vi "CH1_write_byte_data_and_sign_into_mem_no_g_Rev01.vi"(0 "MB data":u8, 1 "UB data":u8, 3 "Address of the sign":string, 4 "USB Interface Name":refnum<visa-resource-name>="COM3", 5 "HB data":u8, 7 "LB data":u8, 8 "MB address":string, 9 "HB address":string, 11 "LB address":string, 12 "Sign Value":dbl, 13 "WRITE DATA":bool, 14 "Input buffer size":u32=16384, 16 "UB address":string, 17 "error in (no error)":errorcluster, 23 "Enable memory wright":bool) -> (18 "Reply 1":string, 19 "Reply 4":string, 20 "MB data string":string, 21 "UB data string":string, 22 "Reply 2":string, 24 "error out":errorcluster, 25 "HB data string":string, 26 "Reply 3":string, 27 "LB data string":string)   [LabVIEW 2012]
panel:
  out "T command Bytes sent 5":dbl
  out "T command Bytes sent 4":dbl
  out "T command Bytes sent 3":dbl
  out "T command Bytes sent 2":dbl
  out "T command Bytes sent":dbl
  out "First 'T' Number of bytes written":dbl
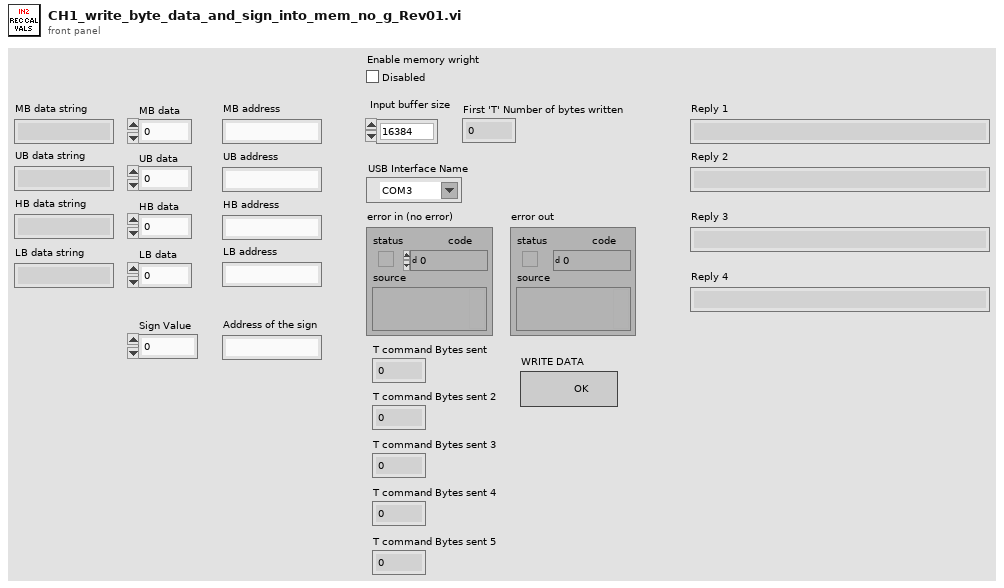
[diagram p1: front panel]
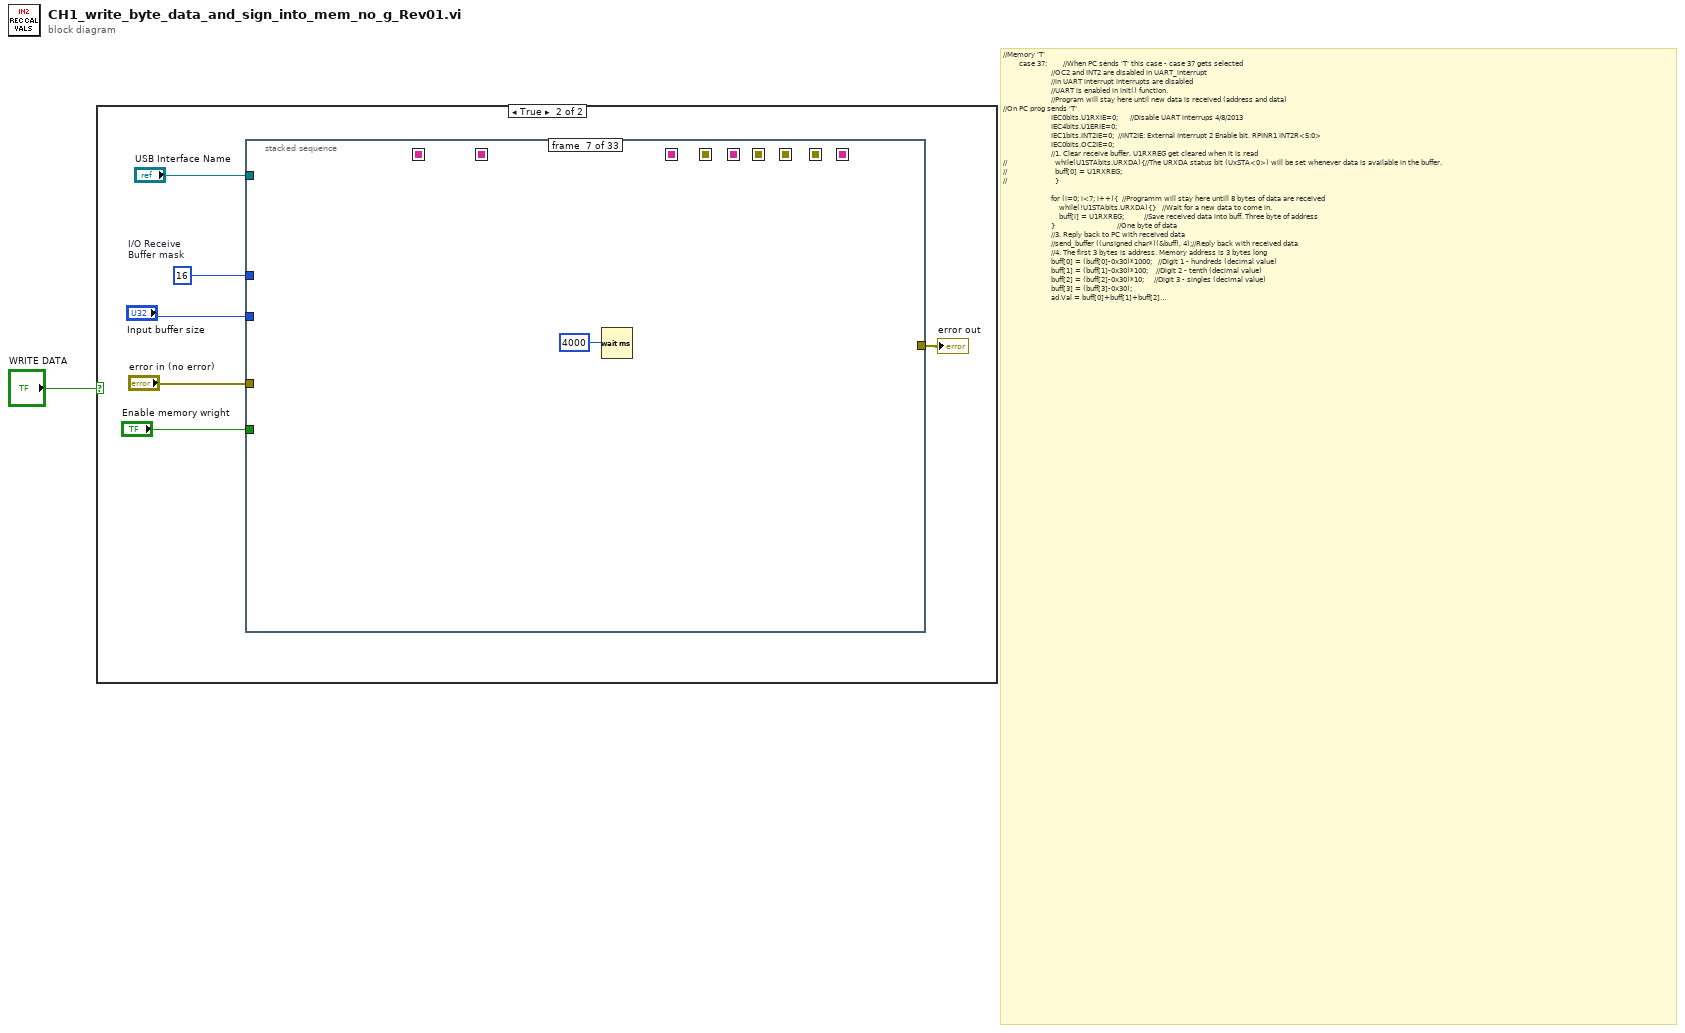
[diagram p0: block diagram]
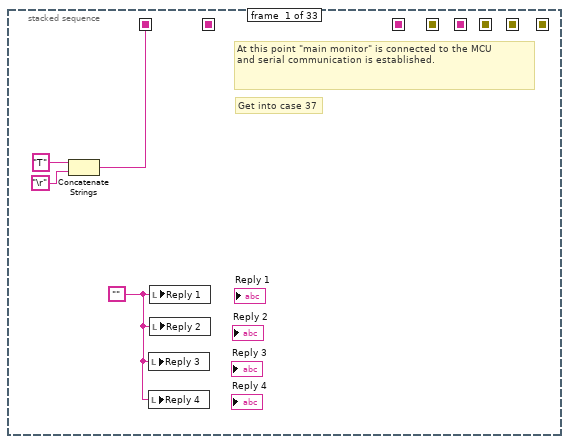
[diagram p3: hidden frame]
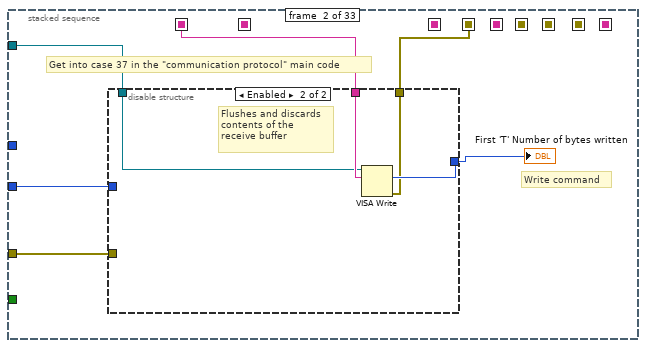
[diagram p4: hidden frame]
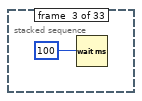
[diagram p6: hidden frame]
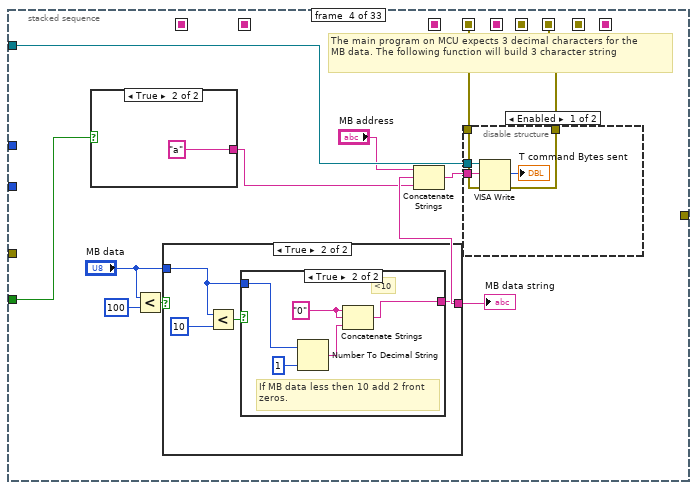
[diagram p7: hidden frame]
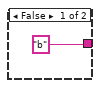
[diagram p8: hidden frame]
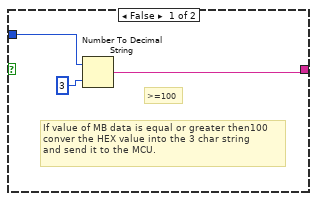
[diagram p9: hidden frame]
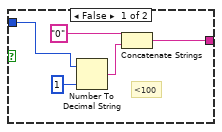
[diagram p10: hidden frame]
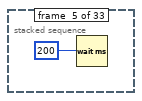
[diagram p12: hidden frame]
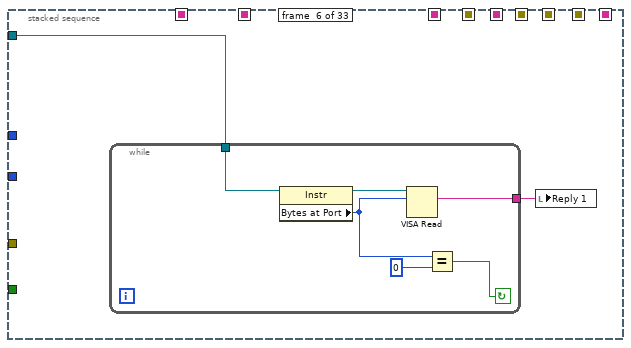
[diagram p13: hidden frame]
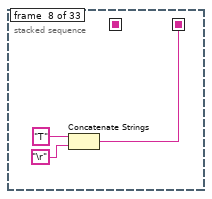
[diagram p14: hidden frame]
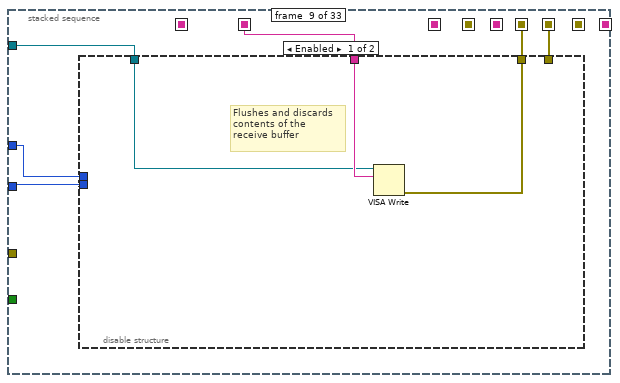
[diagram p15: hidden frame]
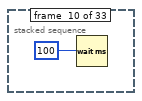
[diagram p17: hidden frame]
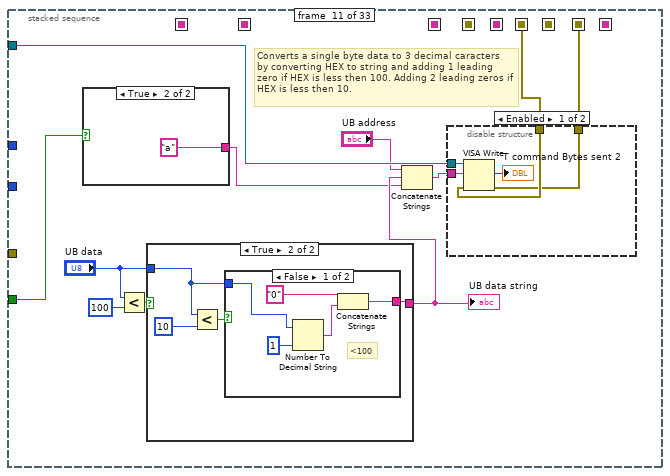
[diagram p18: hidden frame]
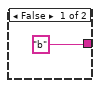
[diagram p19: hidden frame]
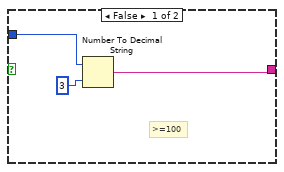
[diagram p20: hidden frame]
diagram:
  # "//Memory 'T'\n        case 37:        //When PC sends 'T' this case - case 37 gets selected\n                        //OC2 and INT2 are disabled in UART_interrupt\n                        //in UART interrupt interrupts are disabled\n                        //UART is enabled in init() function.\n                        //Program will stay here until new data is received (address and data)\n//On PC prog sends 'T'\n                        IEC0bits.U1RXIE=0;      //Disable UART interrups 4/8/2013\n                        IEC4bits.U1ERIE=0;\n                        IEC1bits.INT2IE=0;  //INT2IE: External Interrupt 2 Enable bit. RPINR1 INT2R<5:0>\n                        IEC0bits.OC2IE=0;\n                        //1. Clear receive buffer. U1RXREG get cleared when it is read\n//                        while(U1STAbits.URXDA){//The URXDA status bit (UxSTA<0>) will be set whenever data is available in the buffer.\n//                        buff[0] = U1RXREG;\n//                        }\n\n                        for (i=0; i<7; i++){  //Programm will stay here untill 8 bytes of data are received\n                            while(!U1STAbits.URXDA){}   //Wait for a new data to come in.\n                            buff[i] = U1RXREG;          //Save received data into buff. Three byte of address\n                        }                               //One byte of data\n                        //3. Reply back to PC with received data\n                        //send_buffer ((unsigned char*)(&buff), 4);//Reply back with received data\n                        //4. The first 3 bytes is address. Memory address is 3 bytes long\n                        buff[0] = (buff[0]-0x30)*1000;   //Digit 1 - hundreds (decimal value)\n                        buff[1] = (buff[1]-0x30)*100;    //Digit 2 - tenth (decimal value)\n                        buff[2] = (buff[2]-0x30)*10;     //Digit 3 - singles (decimal value)\n                        buff[3] = (buff[3]-0x30);\n                        ad.Val = buff[0]+buff[1]+buff[2]+buff[3];\n//                        send_char((char) ad.byte.MB);\n//                        send_char((char) ad.byte.UB);\n//                        send_char((char) ad.byte.HB);\n//                        send_char((char) ad.byte.LB); \n                        //5. The last 3 bytes are data\n                        buff[4] = buff[4]-0x30;//Load data. Byte number 4 is the data byte\n                        buff[5] = buff[5]-0x30;\n                        buff[6] = buff[6]-0x30;\n                        data = buff[4]*100+buff[5]*10+buff[6]; //Decimal value of 3 char digits\n                        //send_buffer ((unsigned char*)(&ad), 3);//Send back the received address\n                        //Erase byte by writing FFH into the address\n                        DF_WriteProtectDisable();   //Enable write to memory\n                        DF_IsBusy();                //Wait until the operation is done\n                        DF_WriteByte(ad.Val, data); //Write data into ad\n                        DF_IsBusy();\n                        DF_WriteDisable();          //Disable write\n                        DF_IsBusy();                        \n                        data=DF_ReadByte(ad.Val);     //4/22/13 return BYTE data\n//                       send_char((char) data);              //Read the memory location and reply with previously sent data\n//                        //Memory address for sign\n//                        buff[7] = (buff[7]-0x30)*1000;   //Digit 1 - hundreds (decimal value)\n//                        buff[8] = (buff[8]-0x30)*100;    //Digit 2 - tenth (decimal value)\n//                        buff[9] = (buff[9]-0x30)*10;     //Digit 3 - singles (decimal value)\n//                        buff[10] = (buff[10]-0x30);\n//                        ad.Val = buff[7]+buff[8]+buff[9]+buff[10];\n//                        //sign\n//                        sgn = buff[11];//<12\n                        \n                        selection = 1;\n                        rx_function=0; //4/11/13\n                        IEC0bits.U1RXIE=1;      //Reinable UART interrups\n                        IEC4bits.U1ERIE=1;                        \n                        IEC1bits.INT2IE=1;  //INT2IE: External Interrupt 2 Enable bit. RPINR1 INT2R<5:0>\n                        IEC0bits.OC2IE=1;\n                        \n\n            break;"
  n1 = case shown="True" "WRITE DATA" {
    frame False {
    }
    frame True {
      w5 = u16 16  # I/O Receive Buffer mask
      n2 = stacked-sequence {
        seq-local: [w9 _ _ _ _ _ _ _ _ _ _ _ _ _ _ _ _ _ _ _ _ _ _ _ _ _ _ _ _ _ _ _ _] -> [_ w14 _ _ _ _ _ _ _ _ _ _ _ _ _ _ _ _ _ _ _ _ _ _ _ _ _ _ _ _ _ _ _]
        seq-local: [_ _ _ _ _ _ _ w68 _ _ _ _ _ _ _ _ _ _ _ _ _ _ _ _ _ _ _ _ _ _ _ _ _] -> [_ _ _ _ _ _ _ _ w73 _ _ _ _ _ _ _ _ _ _ _ _ _ _ _ _ _ _ _ _ _ _ _ _]
        seq-local: [_ _ _ _ _ _ _ _ _ _ _ _ _ _ w126 _ _ _ _ _ _ _ _ _ _ _ _ _ _ _ _ _ _] -> [_ _ _ _ _ _ _ _ _ _ _ _ _ _ _ w130 _ _ _ _ _ _ _ _ _ _ _ _ _ _ _ _ _]
        seq-local: [_ _ _ _ _ _ _ _ _ _ _ _ _ _ _ _ _ _ _ _ _ w177 _ _ _ _ _ _ _ _ _ _ _] -> [_ _ _ _ _ _ _ _ _ _ _ _ _ _ _ _ _ _ _ _ _ _ w180 _ _ _ _ _ _ _ _ _ _]
        seq-local: [_ w12 _ _ _ _ _ _ _ _ _ _ _ _ _ _ _ _ _ _ _ _ _ _ _ _ _ _ _ _ _ _ _] -> [_ _ _ w27 _ _ _ _ _ _ _ _ _ _ _ _ _ _ _ _ _ _ _ _ _ _ _ _ _ _ _ _ _]
        seq-local: [_ _ _ w26 _ _ _ _ _ _ _ _ _ _ _ _ _ _ _ _ _ _ _ _ _ _ _ _ _ _ _ _ _] -> [_ _ _ _ _ _ _ _ w72 _ _ _ _ _ _ _ _ _ _ _ _ _ _ _ _ _ _ _ _ _ _ _ _]
        seq-local: [_ _ _ _ _ _ _ _ w71 _ _ _ _ _ _ _ _ _ _ _ _ _ _ _ _ _ _ _ _ _ _ _ _] -> [_ _ _ _ _ _ _ _ _ _ w84 _ _ _ _ _ _ _ _ _ _ _ _ _ _ _ _ _ _ _ _ _ _]
        seq-local: [_ _ _ _ _ _ _ _ _ _ w83 _ _ _ _ _ _ _ _ _ _ _ _ _ _ _ _ _ _ _ _ _ _] -> [_ _ _ _ _ _ _ _ _ _ _ _ _ _ _ w129 _ _ _ _ _ _ _ _ _ _ _ _ _ _ _ _ _]
        seq-local: [_ _ _ _ _ _ _ _ _ _ _ _ _ _ _ _ _ _ _ _ _ _ _ _ _ _ _ _ w231 _ _ _ _] -> [_ _ _ _ _ _ _ _ _ _ _ _ _ _ _ _ _ _ _ _ _ _ _ _ _ _ _ _ _ w234 _ _ _]
        tunnel: "USB Interface Name" -> [_ w17 _ w32 _ w60 _ _ w76 _ w86 _ w118 _ _ w133 _ w140 _ w169 _ _ w184 _ w193 _ w223 _ _ w238 _ w251 _]
        tunnel: "error in (no error)" -> [_ w16 _ _ _ _ _ _ _ _ _ _ _ _ _ _ _ _ _ _ _ _ w182 _ _ _ _ _ _ w235 _ _ _]
        tunnel: "Input buffer size" -> [_ w15 _ _ _ _ _ _ w75 _ _ _ _ _ _ w131 _ _ _ _ _ _ w183 _ _ _ _ _ _ w236 _ _ _]
        tunnel: w5 -> [_ _ _ _ _ _ _ _ w74 _ _ _ _ _ _ w132 _ _ _ _ _ _ w181 _ _ _ _ _ _ w237 _ _ _]
        tunnel: [_ _ _ _ _ _ _ _ _ _ _ _ _ _ _ _ _ _ _ _ _ _ _ _ w191 _ _ _ _ _ _ _ _] -> w4
        tunnel: "Enable memory wright" -> [_ _ _ w24 _ _ _ _ _ _ w82 _ _ _ _ _ _ w138 _ _ _ _ _ _ w189 _ _ _ _ _ _ w243 _]
        frame #0 {
          w8 = ""
          # "At this point \"main monitor\" is connected to the MCU\nand serial communication is established."
          # "Get into case 37"
          n3 = Concatenate Strings("T", "\r") -> (w9:string)
          n4 = local write "Reply 3"(w8) -> ()
          n5 = local write "Reply 4"(w8) -> ()
          n6 = local write "Reply 1"(w8) -> ()
          n7 = local write "Reply 2"(w8) -> ()
        }
        frame #1 {
          # "Get into case 37 in the \"communication protocol\" main code"
          # "Write command"
          n8 = disable-structure shown="Enabled" {
            disable-tunnel: w15 -> [_ _]
            disable-tunnel: w14 -> [_ w21]
            disable-tunnel: w17 -> [_ w18]
            disable-tunnel: w16 -> [_ _]
            disable-tunnel: [_ w20] -> w13
            disable-tunnel: [_ w19] -> w12
            frame Disabled {
            }
            frame Enabled {
              # "Flushes and discards \ncontents of the \nreceive buffer"
              n9 = VISA Write(VISA resource name=w18, write buffer=w21) -> (return count=w20:u32, error out=w19:errorcluster)  [unwired: 1 in, 1 out]
            }
          }
          "First 'T' Number of bytes written" <- w13
        }
        frame #2 {
          n10 = Wait (ms)(milliseconds to wait=100) -> ()  [unwired: 1 out]
        }
        frame #3 {
          # "The main program on MCU expects 3 decimal characters for the \nMB data. The following function will build 3 character string"
          n11 = case shown="True" w24 {
            tunnel: ["b" "a"] -> w23
            frame False {
            }
            frame True {
            }
          }
          n12 = Less?(x="MB data", y=100) -> (x < y?=w31:bool)
          n13 = case shown="True" w31 {
            tunnel: [w38 w39] -> w28
            tunnel: "MB data" -> [w36 w40]
            frame False {
              # "If value of MB data is equal or greater then100\nconver the HEX value into the 3 char string \nand send it to the MCU."
              # ">=100"
              n14 = Number To Decimal String(number=w36, width (-)=3) -> (decimal integer string=w38:string)
            }
            frame True {
              n15 = Less?(x=w40, y=10) -> (x < y?=w42:bool)
              n16 = case shown="True" w42 {
                tunnel: w40 -> [w44 w48]
                tunnel: [w43 w49] -> w39
                frame False {
                  # "<100"
                  n17 = Number To Decimal String(number=w44, width (-)=1) -> (decimal integer string=w45:string)
                  n18 = Concatenate Strings("0", w45) -> (w43:string)
                }
                frame True {
                  w50 = "0"
                  # "If MB data less then 10 add 2 front\nzeros."
                  # "<10"
                  n19 = Number To Decimal String(number=w48, width (-)=1) -> (decimal integer string=w51:string)
                  n20 = Concatenate Strings(w50, w50, w51) -> (w49:string)
                }
              }
            }
          }
          "MB data string" <- w28
          n21 = Concatenate Strings("MB address", w28, w23) -> (w33:string)
          n22 = disable-structure shown="Enabled" {
            disable-tunnel: w33 -> [w56 _]
            disable-tunnel: w32 -> [w55 _]
            disable-tunnel: w27 -> [w54 _]
            disable-tunnel: [w53 _] -> w26
            frame Enabled {
              n23 = VISA Write(VISA resource name=w55, write buffer=w56, error in (no error)=w54) -> (return count=→"T command Bytes sent":u32, error out=w53:errorcluster)  [unwired: 1 out]
            }
            frame Disabled {
            }
          }
        }
        frame #4 {
          n24 = Wait (ms)(milliseconds to wait=200) -> ()  [unwired: 1 out]
        }
        frame #5 {
          n25 = while {
            tunnel: w60 -> [w62]
            tunnel: [w61] -> w59
            stop <- w63 continue-if-true
            n26 = property class="Instr"(reference=w62) -> (reference out=w66:refnum<visa-resource-name>, "Bytes at Port"=w65:u32)  [unwired: 1 in, 1 out]
            n27 = VISA Read(VISA resource name=w66, byte count=w65) -> (read buffer=w61:string)  [unwired: 1 in, 3 out]
            n28 = Equal?(x=w65, y=0) -> (x = y?=w63:bool)
          }
          n29 = local write "Reply 1"(w59) -> ()
        }
        frame #6 {
          n30 = Wait (ms)(milliseconds to wait=4000) -> ()  [unwired: 1 out]
        }
        frame #7 {
          n31 = Concatenate Strings("T", "\r") -> (w68:string)
        }
        frame #8 {
          n32 = disable-structure shown="Enabled" {
            disable-tunnel: w76 -> [w77 _]
            disable-tunnel: w75 -> [_ _]
            disable-tunnel: w74 -> [_ _]
            disable-tunnel: w73 -> [w79 _]
            disable-tunnel: w72 -> [_ _]
            disable-tunnel: [w78 _] -> w71
            frame Enabled {
              # "Flushes and discards \ncontents of the \nreceive buffer"
              n33 = VISA Write(VISA resource name=w77, write buffer=w79) -> (error out=w78:errorcluster)  [unwired: 1 in, 2 out]
            }
            frame Disabled {
            }
          }
        }
        frame #9 {
          n34 = Wait (ms)(milliseconds to wait=100) -> ()  [unwired: 1 out]
        }
        frame #10 {
          # "Converts a single byte data to 3 decimal caracters\nby converting HEX to string and adding 1 leading zero if HEX is less then 100. Adding 2 leading zeros if HEX is less then 10."
          n35 = case shown="True" w82 {
            tunnel: ["b" "a"] -> w81
            frame False {
            }
            frame True {
            }
          }
          n36 = Less?(x="UB data", y=100) -> (x < y?=w90:bool)
          n37 = case shown="True" w90 {
            tunnel: [w96 w97] -> w87
            tunnel: "UB data" -> [w94 w98]
            frame False {
              # ">=100"
              n38 = Number To Decimal String(number=w94, width (-)=3) -> (decimal integer string=w96:string)
            }
            frame True {
              n39 = Less?(x=w98, y=10) -> (x < y?=w100:bool)
              n40 = case shown="False" w100 {
                tunnel: w98 -> [w102 w106]
                tunnel: [w101 w107] -> w97
                frame False {
                  # "<100"
                  n41 = Number To Decimal String(number=w102, width (-)=1) -> (decimal integer string=w103:string)
                  n42 = Concatenate Strings("0", w103) -> (w101:string)
                }
                frame True {
                  w108 = "0"
                  # "<10"
                  n43 = Number To Decimal String(number=w106, width (-)=1) -> (decimal integer string=w109:string)
                  n44 = Concatenate Strings(w108, w108, w109) -> (w107:string)
                }
              }
            }
          }
          "UB data string" <- w87
          n45 = Concatenate Strings("UB address", w87, w81) -> (w91:string)
          n46 = disable-structure shown="Enabled" {
            disable-tunnel: w91 -> [w114 _]
            disable-tunnel: w86 -> [w113 _]
            disable-tunnel: w84 -> [w112 _]
            disable-tunnel: [w111 _] -> w83
            frame Enabled {
              n47 = VISA Write(VISA resource name=w113, write buffer=w114, error in (no error)=w112) -> (return count=→"T command Bytes sent 2":u32, error out=w111:errorcluster)  [unwired: 1 out]
            }
            frame Disabled {
            }
          }
        }
        frame #11 {
          n48 = Wait (ms)(milliseconds to wait=200) -> ()  [unwired: 1 out]
        }
        frame #12 {
          n49 = while {
            tunnel: w118 -> [w120]
            tunnel: [w119] -> w117
            stop <- w121 continue-if-true
            n50 = property class="Instr"(reference=w120) -> (reference out=w124:refnum<visa-resource-name>, "Bytes at Port"=w123:u32)  [unwired: 1 in, 1 out]
            n51 = VISA Read(VISA resource name=w124, byte count=w123) -> (read buffer=w119:string)  [unwired: 1 in, 3 out]
            n52 = Equal?(x=w123, y=0) -> (x = y?=w121:bool)
          }
          n53 = local write "Reply 2"(w117) -> ()
        }
        frame #13 {
          n54 = Wait (ms)(milliseconds to wait=4000) -> ()  [unwired: 1 out]
        }
        frame #14 {
          n55 = Concatenate Strings("T", "\r") -> (w126:string)
        }
        frame #15 {
          n56 = disable-structure shown="Enabled" {
            disable-tunnel: w133 -> [w134 _]
            disable-tunnel: w132 -> [_ _]
            disable-tunnel: w131 -> [_ _]
            disable-tunnel: w130 -> [w135 _]
            disable-tunnel: w129 -> [_ _]
            frame Enabled {
              # "Flushes and discards \ncontents of the \nreceive buffer"
              n57 = VISA Write(VISA resource name=w134, write buffer=w135) -> ()  [unwired: 1 in, 3 out]
            }
            frame Disabled {
            }
          }
        }
        frame #16 {
          n58 = Wait (ms)(milliseconds to wait=1000) -> ()  [unwired: 1 out]
        }
        frame #17 {
          # "Converts a single byte data to 3 decimal caracters\nby converting HEX to string and adding 1 leading zero if HEX is less then 100. Adding 2 leading zeros if HEX is less then 10."
          n59 = case shown="True" w138 {
            tunnel: ["b" "a"] -> w137
            frame False {
            }
            frame True {
            }
          }
          n60 = Less?(x="HB data", y=100) -> (x < y?=w144:bool)
          n61 = case shown="True" w144 {
            tunnel: [w150 w151] -> w141
            tunnel: "HB data" -> [w148 w152]
            frame False {
              # ">=100"
              n62 = Number To Decimal String(number=w148, width (-)=3) -> (decimal integer string=w150:string)
            }
            frame True {
              n63 = Less?(x=w152, y=10) -> (x < y?=w154:bool)
              n64 = case shown="False" w154 {
                tunnel: w152 -> [w156 w160]
                tunnel: [w155 w161] -> w151
                frame False {
                  # "<100"
                  n65 = Number To Decimal String(number=w156, width (-)=1) -> (decimal integer string=w157:string)
                  n66 = Concatenate Strings("0", w157) -> (w155:string)
                }
                frame True {
                  w162 = "0"
                  # "<10"
                  n67 = Number To Decimal String(number=w160, width (-)=1) -> (decimal integer string=w163:string)
                  n68 = Concatenate Strings(w162, w162, w163) -> (w161:string)
                }
              }
            }
          }
          "HB data string" <- w141
          n69 = Concatenate Strings("HB address", w141, w137) -> (w145:string)
          n70 = disable-structure shown="Enabled" {
            disable-tunnel: w145 -> [w166 _]
            disable-tunnel: w140 -> [w165 _]
            frame Enabled {
              n71 = VISA Write(VISA resource name=w165, write buffer=w166) -> (return count=→"T command Bytes sent 3":u32)  [unwired: 1 in, 2 out]
            }
            frame Disabled {
            }
          }
        }
        frame #18 {
          n72 = Wait (ms)(milliseconds to wait=100) -> ()  [unwired: 1 out]
        }
        frame #19 {
          n73 = while {
            tunnel: w169 -> [w171]
            tunnel: [w170] -> _
            stop <- w172 continue-if-true
            n74 = property class="Instr"(reference=w171) -> (reference out=w175:refnum<visa-resource-name>, "Bytes at Port"=w174:u32)  [unwired: 1 in, 1 out]
            n75 = VISA Read(VISA resource name=w175, byte count=w174) -> (read buffer=w170:string)  [unwired: 1 in, 3 out]
            n76 = Equal?(x=w174, y=0) -> (x = y?=w172:bool)
          }
        }
        frame #20 {
          n77 = Wait (ms)(milliseconds to wait=3000) -> ()  [unwired: 1 out]
        }
        frame #21 {
          # "Get into case 37"
          n78 = Concatenate Strings("T", "\r") -> (w177:string)
        }
        frame #22 {
          # "Get into case 37 in the communication protocol"
          # "Write command"
          n79 = disable-structure shown="Enabled" {
            disable-tunnel: w183 -> [_ _]
            disable-tunnel: w180 -> [w187 _]
            disable-tunnel: w184 -> [w185 _]
            disable-tunnel: w182 -> [_ _]
            disable-tunnel: [w186 _] -> _
            disable-tunnel: w181 -> [_ _]
            frame Enabled {
              # "Flushes and discards \ncontents of the \nreceive buffer"
              n80 = VISA Write(VISA resource name=w185, write buffer=w187) -> (return count=w186:u32)  [unwired: 1 in, 2 out]
            }
            frame Disabled {
            }
          }
        }
        frame #23 {
          n81 = Wait (ms)(milliseconds to wait=1000) -> ()  [unwired: 1 out]
        }
        frame #24 {
          # "The main program on MCU expects 3 decimal characters for the \nMB data. The following function will build 3 character string"
          n82 = case shown="True" w189 {
            tunnel: ["b" "a"] -> w190
            frame False {
            }
            frame True {
            }
          }
          n83 = Less?(x="LB data", y=100) -> (x < y?=w197:bool)
          n84 = case shown="True" w197 {
            tunnel: [w203 w204] -> w194
            tunnel: "LB data" -> [w201 w205]
            frame False {
              # ">=100"
              n85 = Number To Decimal String(number=w201, width (-)=3) -> (decimal integer string=w203:string)
            }
            frame True {
              n86 = Less?(x=w205, y=10) -> (x < y?=w207:bool)
              n87 = case shown="True" w207 {
                tunnel: w205 -> [w209 w213]
                tunnel: [w208 w214] -> w204
                frame False {
                  # "<100"
                  n88 = Number To Decimal String(number=w209, width (-)=1) -> (decimal integer string=w210:string)
                  n89 = Concatenate Strings("0", w210) -> (w208:string)
                }
                frame True {
                  w215 = "0"
                  # "<10"
                  n90 = Number To Decimal String(number=w213, width (-)=1) -> (decimal integer string=w216:string)
                  n91 = Concatenate Strings(w215, w215, w216) -> (w214:string)
                }
              }
            }
          }
          "LB data string" <- w194
          n92 = Concatenate Strings("LB address", w194, w190) -> (w198:string)
          n93 = disable-structure shown="Enabled" {
            disable-tunnel: w198 -> [w220 _]
            disable-tunnel: w193 -> [w219 _]
            disable-tunnel: [w218 _] -> w191
            frame Enabled {
              n94 = VISA Write(VISA resource name=w219, write buffer=w220) -> (return count=→"T command Bytes sent 4":u32, error out=w218:errorcluster)  [unwired: 1 in, 1 out]
            }
            frame Disabled {
            }
          }
        }
        frame #25 {
          n95 = Wait (ms)(milliseconds to wait=100) -> ()  [unwired: 1 out]
        }
        frame #26 {
          n96 = while {
            tunnel: w223 -> [w225]
            tunnel: [w224] -> _
            stop <- w226 continue-if-true
            n97 = property class="Instr"(reference=w225) -> (reference out=w229:refnum<visa-resource-name>, "Bytes at Port"=w228:u32)  [unwired: 1 in, 1 out]
            n98 = VISA Read(VISA resource name=w229, byte count=w228) -> (read buffer=w224:string)  [unwired: 1 in, 3 out]
            n99 = Equal?(x=w228, y=0) -> (x = y?=w226:bool)
          }
        }
        frame #27 {
          n100 = Wait (ms)(milliseconds to wait=3000) -> ()  [unwired: 1 out]
        }
        frame #28 {
          n101 = Concatenate Strings("T", "\r") -> (w231:string)
        }
        frame #29 {
          # "Get into case 37 in the communication protocol"
          # "Write command"
          n102 = disable-structure shown="Enabled" {
            disable-tunnel: w236 -> [_ _]
            disable-tunnel: w234 -> [w241 _]
            disable-tunnel: w238 -> [w239 _]
            disable-tunnel: w235 -> [_ _]
            disable-tunnel: [w240 _] -> _
            disable-tunnel: w237 -> [_ _]
            frame Enabled {
              # "Flushes and discards \ncontents of the \nreceive buffer"
              n103 = VISA Write(VISA resource name=w239, write buffer=w241) -> (return count=w240:u32)  [unwired: 1 in, 2 out]
            }
            frame Disabled {
            }
          }
        }
        frame #30 {
          n104 = Wait (ms)(milliseconds to wait=1000) -> ()  [unwired: 1 out]
        }
        frame #31 {
          w248 = "0"
          # "<10"
          n105 = case shown="True" w243 {
            tunnel: ["b" "a"] -> w244
            frame False {
            }
            frame True {
            }
          }
          n106 = Number To Decimal String(number="Sign Value", width (-)=1) -> (decimal integer string=w249:string)
          n107 = Concatenate Strings(w248, w248, w249) -> (w246:string)
          n108 = Concatenate Strings("Address of the sign", w246, w244) -> (w252:string)
          n109 = disable-structure shown="Enabled" {
            disable-tunnel: w252 -> [w257 _]
            disable-tunnel: w251 -> [w256 _]
            disable-tunnel: [w255 _] -> _
            frame Enabled {
              n110 = VISA Write(VISA resource name=w256, write buffer=w257) -> (return count=→"T command Bytes sent 5":u32, error out=w255:errorcluster)  [unwired: 1 in, 1 out]
            }
            frame Disabled {
            }
          }
        }
        frame #32 {
          n111 = Wait (ms)(milliseconds to wait=3000) -> ()  [unwired: 1 out]
        }
      }
      "error out" <- w4
    }
  }
